vi "_USB_CAN_DEBUG_LOG_OUT_.vi"(7 "Trans?":bool, 8 "id":u32, 9 "Info":string, 10 "Edata":i64[](array[numeric]), 11 "TIME":timestamp) -> ()   [LabVIEW 2011]
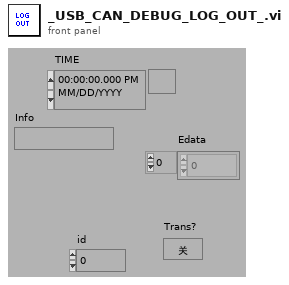
[diagram p1: front panel]
types:
  T1 = enum16{"open", "replace", "create", "open or create", "replace or create", "replace or create with confirmation"}
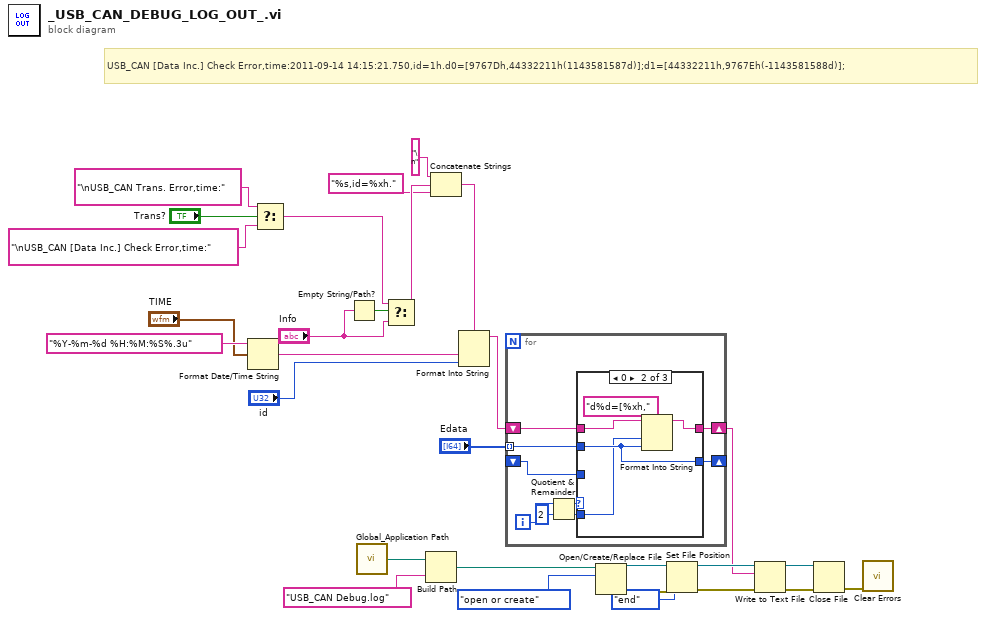
[diagram p0: block diagram]
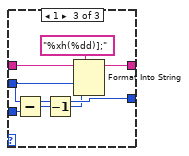
[diagram p3: hidden frame]
diagram:
  # "USB_CAN [Data Inc.] Check Error,time:2011-09-14 14:15:21.750,id=1h.d0=[9767Dh,44332211h(1143581587d)];d1=[44332211h,9767Eh(-1143581588d)];"
  n1 = Format Date/Time String(time format string (%c)="%Y-%m-%d %H:%M:%S%.3u" ("时间格式字符串(%c)"), seconds (now)="TIME") -> (date/time string=w27:string)  [unwired: 1 in]
  n2 = Select(t="\nUSB_CAN Trans. Error,time:" ("格式字符串"), s="Trans?", f="\nUSB_CAN [Data Inc.] Check Error,time:" ("格式字符串")) -> (s? t:f=w2:string)
  n3 = Empty String/Path?(string/path="Info") -> (empty?=w7:bool)
  n4 = call "Global_Application Path.vi"() -> ("程序路径"=w8:path)  [unwired: 1 in]
  n5 = Select(t=w2, s=w7, f="Info") -> (s? t:f=w5:string)
  n6 = Build Path(base path=w8, name or relative path="USB_CAN Debug.log" ("名称或相对路径")) -> (appended path=w24:path)
  n7 = Concatenate Strings("\n" ("字符串"), w5, "%s,id=%xh." ("字符串")) -> (w3:string)
  n8 = Format Into String(format string=w3, w27, "id") -> (resulting string=w14:string)  [unwired: 2 in, 1 out]
  n9 = for {
    tunnel: "Edata" -> [w33] mode=indexing
    shift-right: [w37] -> w13
    shift-left: w14 -> [w38]
    shift-right: [w32] -> _
    shift-left: _ -> [w31]
    i -> [w36]
    n10 = Quotient & Remainder(x=w36, y=2) -> (x-y*floor(x/y)=w34:i32, floor(x/y)=w30:i32)
    n11 = case shown="0" w34 {
      tunnel: w38 -> [w40 w45 w52]
      tunnel: [w40 w44 w51] -> w37
      tunnel: w33 -> [w39 w42 w48]
      tunnel: [w39 w42 w48] -> w32
      tunnel: w31 -> [_ _ w47]
      tunnel: w30 -> [_ w41 _]
      frame -1, Default {
      }
      frame 0 {
        n12 = Format Into String(format string="d%d=[%xh," ("格式字符串"), initial string=w45, w41, w42) -> (resulting string=w44:string)  [unwired: 1 in, 1 out]
      }
      frame 1 {
        n13 = Subtract(x=w48, y=w47) -> (x-y=w49:i64)
        n14 = Decrement(x=w49) -> (x-1=w46:i64)
        n15 = Format Into String(format string="%xh(%dd)];" ("格式字符串"), initial string=w52, w48, w46) -> (resulting string=w51:string)  [unwired: 1 in, 1 out]
      }
    }
  }
  n16 = Open/Create/Replace File(file path (use dialog)=w24, operation (0:open)=T1."open or create" ("操作(0:open)")) -> (refnum out=w22:refnum<file>, error out=w21:errorcluster)  [unwired: 4 in, 1 out]
  n17 = Set File Position(refnum=w22, from (0:start)=enum16{"start", "end", "current"}."end" ("自（0:起始）"), error in=w21) -> (refnum out=w19:refnum<file>, error out=w18:errorcluster)  [unwired: 1 in]
  n18 = Write to Text File(file (use dialog)=w19, text=w13, error in=w18) -> (refnum out=w16:refnum<file>, error out=w17:errorcluster)  [unwired: 1 in, 1 out]
  n19 = Close File(refnum=w16, error in=w17) -> (error out=w12:errorcluster)  [unwired: 1 out]
  n20 = call <vilib>:"Clear Errors.vi"("error in (no error)"=w12) -> ()  [unwired: 6 in, 1 out]
